vi "Refresh SRs.vi"(8 "error in":errorcluster, 11 "Data Loop Data in":T1) -> (0 "error out":errorcluster, 3 "Data Loop Data out":T1)   [LabVIEW 2018]
uses:
  Type Defs/FGV States.ctl
  Type Defs/Screenpop Loop Data.ctl
  Support/Message Queue/Message Cluster.ctl
  Support/Message Queue/Message Queue.lvlib
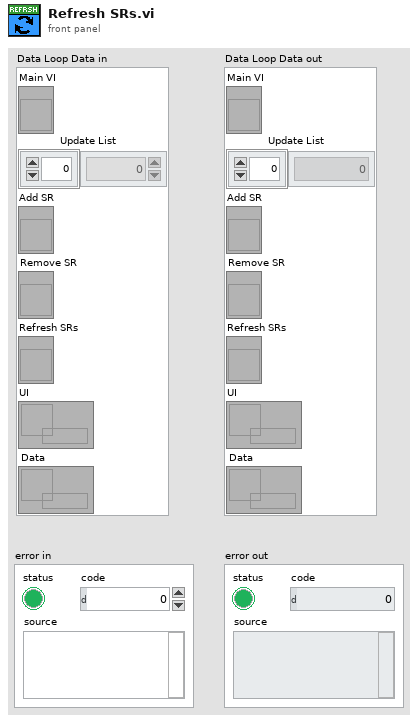
[diagram p1: front panel]
types:
  T1 = typedef "Screenpop Loop Data.ctl" = cluster{"Main VI":refnum<vi>, "Update List":i32[], "Add SR":refnum<vi>, "Remove SR":refnum<vi>, "Refresh SRs":refnum<vi>, "UI":refnum<queue>, "Data":refnum<queue>}
  T2 = typedef "FGV States.ctl" = enum16{"Initialize", "Merge", "Write", "Read", "Clear"}
  T3 = typedef "SR Cluster.ctl" = cluster{"Color":u32, "SR Number":i32, "SR Status":T4, "Name":string, "Summary":string, "Last Updated":timestamp, "SR Type":string, "Service Level":string, "Days Open":dbl, "Creation Date":timestamp, "Owner":string, "Note":string}
  T4 = typedef "SR Status.ctl" = enum16{"Caller Abandoned", "Created in Error", "Expired", "Forum Resolved AE", "Forum Resolved Customer", "IN WORK", "IN WORK Collab with AES", "IN WORK Collab with PSE", "IN WORK Collab with SE", "IN WORK Customer Added Note", "IN WORK Escalation", "IN WORK Wait on Customer", "Open", "Potentially Resolved", "Presumed Resolved", "RMA Approved for Return", "RMA Closed", "RMA Closed - DOA", "RMA In Progress", "RMA Open", "RMA Waiting on Customer", "Resolved", "Passed Off"}
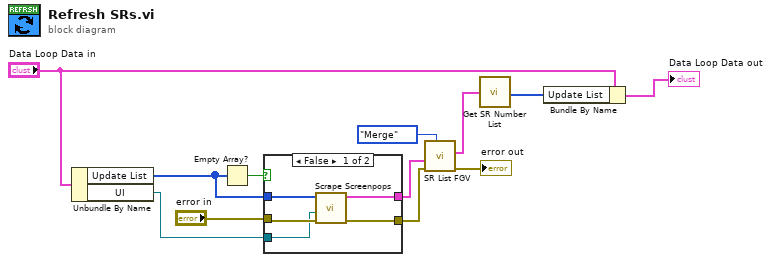
[diagram p0: block diagram]
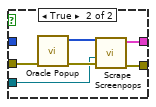
[diagram p2: hidden frame]
diagram:
  n1 = Unbundle By Name("Data Loop Data in") -> ("Update List"=w9:i32[], "UI"=w6:refnum<queue>)
  n2 = Empty Array?(array=w9) -> (empty?=w10:bool)
  n3 = case shown="False" w10 {
    tunnel: [w15 w23] -> w2
    tunnel: [w16 w22] -> w4
    tunnel: w9 -> [w17 _]
    tunnel: "error in" -> [w14 w19]
    tunnel: w6 -> [w13 w18]
    frame False {
      n4 = call "Scrape Screenpops.vi"("error in"=w14, "UI"=w13, "SR number list in"=w17) -> ("error out"=w15:errorcluster, "sr clusters out"=w16:T3[])  [unwired: 7 in]
    }
    frame True {
      n5 = call "Oracle Popup.vi"("error in"=w19) -> ("error out"=w20:errorcluster, "SR array out"=w21:i32[])  [unwired: 9 in]
      n6 = call "Scrape Screenpops.vi"("error in"=w20, "UI"=w18, "SR number list in"=w21) -> ("error out"=w23:errorcluster, "sr clusters out"=w22:T3[])  [unwired: 7 in]
    }
  }
  n7 = call "SR List FGV.vi"("Operation"=FGV_States."Merge", "Error In"=w2, "Input"=w4) -> ("Error Out"=→"error out":errorcluster, "list out"=w3:T3[])  [unwired: 7 in]
  n8 = call "Get SR Number List.vi"("list in"=w3) -> ("SR number array out"=w7:i32[])  [unwired: 4 in]
  n9 = Bundle By Name(cluster="Data Loop Data in", "Update List"=w7) -> (→"Data Loop Data out":T1)
